vi "Refresh Host Parameters.vi"(8 "error in (no error)":errorcluster, 10 "Async Parameter Array":dbl[](array[numeric]), 11 "State Vars.CompiledSettings.RunTimeParameterChannels":T1[](array[typedef]) {"Channel Data Reference" format="%.0x"}) -> (0 "error out":errorcluster, 2 "Updated Async Parameter Array":dbl[](array[numeric]))   [LabVIEW 2014, in "Waveform-Processing-Custom-Device Engine.lvlib"]
uses:
  Waveform-Processing-Custom-Device Engine.lvlib
  Shared/VSChannel.ctl
  <vilib>/NI Veristand/Custom Device API/Data Reference.ctl
  <vilib>/NI Veristand/Custom Device API/Custom Device API.lvlib
  Shared/Waveform-Processing-Custom-Device Shared.lvlib
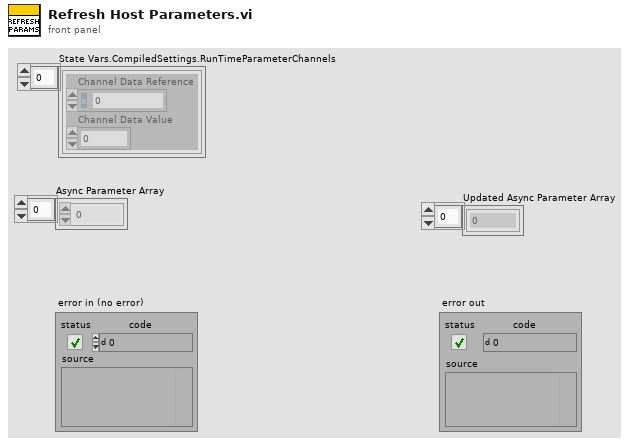
[diagram p1: front panel]
types:
  T1 = typedef "Waveform-Processing-Custom-Device Shared.lvlib/VSChannel.ctl" = cluster{"Channel Data Reference":T2, "Channel Data Value":dbl}
  T2 = typedef "Custom Device API.lvlib/Data Reference.ctl" = i32
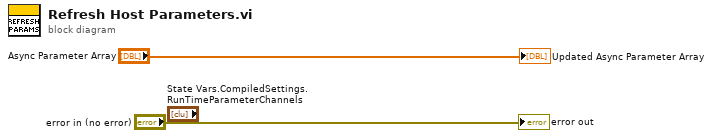
[diagram p0: block diagram]
diagram:
  "error out" <- "error in (no error)"
  "Updated Async Parameter Array" <- "Async Parameter Array"
